vi "Row_Sum and Col_Sum Plots.vi"(0 "Row_Sum":i16[](array[numeric]), 1 "Col_Sum":i16[](array[numeric]), 2 "Cum_Col_Sum":i16[](array[numeric]), 5 "error in (no error)":errorcluster, 7 "cumulative?":bool) -> (14 "Row_Sum Plot":cluster{"X":i16[], "Y":i32[]}[](array[cluster]), 15 "Col_Sum Plot":cluster{"X":i32[], "Y":i16[]}, 19 "error out":errorcluster)   [LabVIEW 2015]
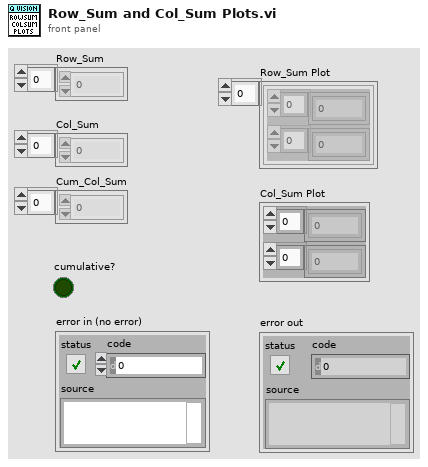
[diagram p1: front panel]
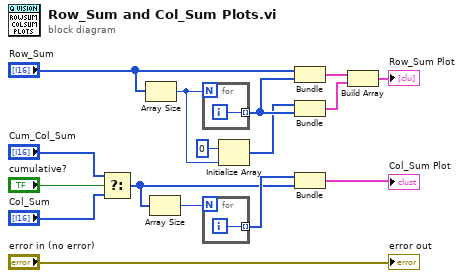
[diagram p0: block diagram]
diagram:
  n1 = Select(t="Cum_Col_Sum", s="cumulative?", f="Col_Sum") -> (s? t:f=w2:i16[])
  n2 = Array Size(array="Row_Sum") -> (size(s)=w11:i32)
  n3 = Array Size(array=w2) -> (size(s)=w7:i32)
  n4 = for {
    N: w11 -> [_]
    tunnel: [w17] -> w12 mode=indexing
    i -> [w17]
  }
  n5 = for {
    N: w7 -> [_]
    tunnel: [w18] -> w10 mode=indexing
    i -> [w18]
  }
  n6 = Initialize Array(i16 0 ("element"), w11) -> (w9:i16[])
  n7 = Bundle("Row_Sum"="Row_Sum", w12) -> (w14:cluster{"Row_Sum":i16[], i32[]})  [unwired: 1 in]
  n8 = Bundle(w9, w12) -> (w15:cluster{i16[], i32[]})  [unwired: 1 in]
  n9 = Bundle(w10, "Col_Sum"=w2) -> (→"Col_Sum Plot":cluster{i32[], "Col_Sum":i16[]})  [unwired: 1 in]
  n10 = Build Array(w14, w15) -> (→"Row_Sum Plot":cluster{"Row_Sum":i16[], i32[]}[])
  "error out" <- "error in (no error)"
